vi "FMA1600A Main.vi"() -> ()   [LabVIEW 2016]
uses:
  Type Definitions/FMA1600A Gas Type.ctl
  Type Definitions/FMA1600A Commands.ctl
  Alicat Gas Meter Driver/Sub-VIs/Data Cluster.ctl
  <vilib>/Utility/file.llb/Write To Spreadsheet File (string).vi
  <vilib>/Utility/file.llb/Write Delimited Spreadsheet (string).vi
panel:
  out "Data Cluster":T1
  in  "Use Data Save":bool
  in  "Scan Rate (mS)":u32=1000
  in  "file path (dialog if empty)":path=path "C:/Data/FMA1600A.csv"
  in  "Tab Control":enum32{"Page 1", "Page 2"}(tab)
  out "error out":errorcluster
  in  "Unit ID":string="A"
  in  "FMA1600A Commands":T2="*@="
  in  "Gas Type":T3="2"
  in  "stop":bool
  in  "VISA resource name":refnum<visa-resource-name>="COM3"
  # "Totalizer Timer"
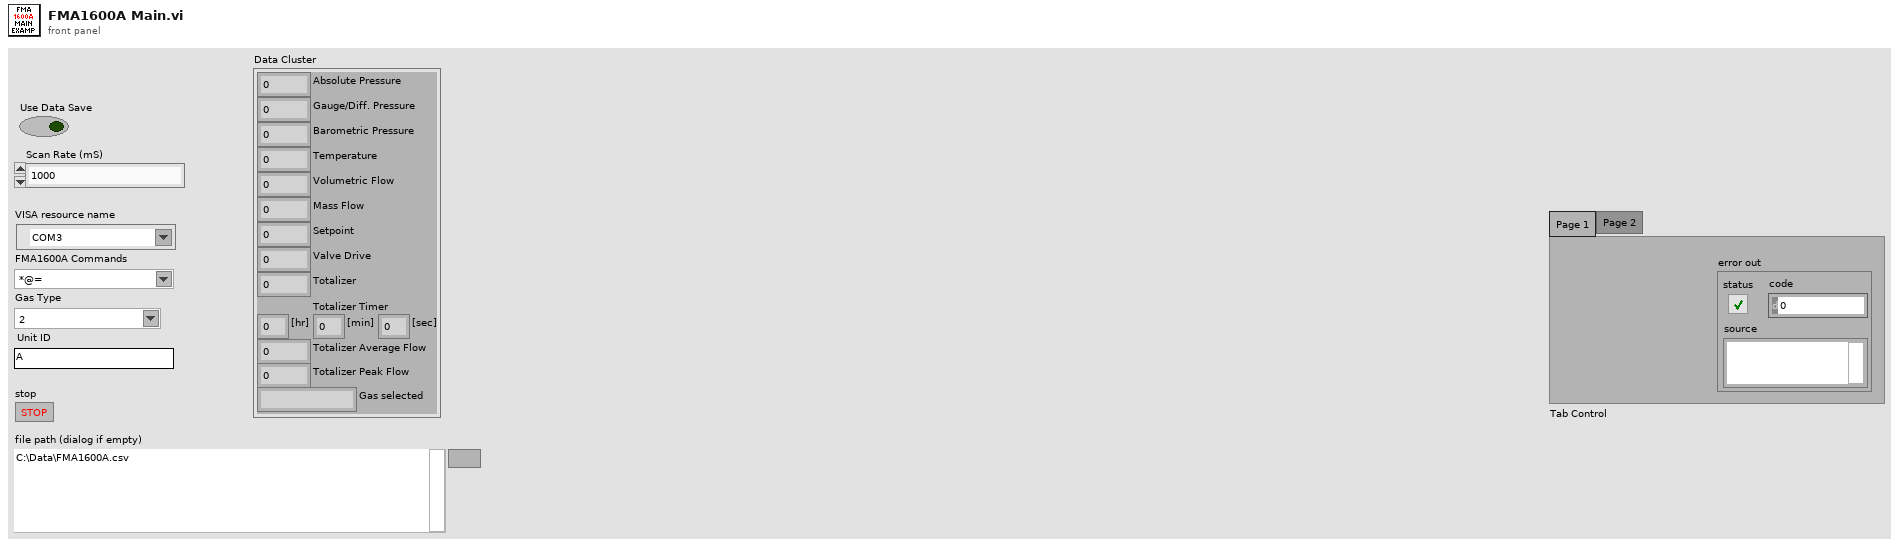
[diagram p1: front panel]
types:
  T1 = typedef "Data Cluster.ctl" = cluster{"Absolute Pressure":dbl, "Gauge/Diff. Pressure":dbl, "Barometric Pressure":dbl, "Temperature":dbl, "Volumetric Flow":dbl, "Mass Flow":dbl, "Setpoint":dbl, "Valve Drive":dbl, "Totalizer":dbl, "[hr]":dbl, "[min]":dbl, "[sec]":dbl, "Totalizer Average Flow":dbl, "Totalizer Peak Flow":dbl, "Gas selected":string}
  T2 = typedef "FMA1600A Commands.ctl" = string
  T3 = typedef "FMA1600A Gas Type.ctl" = string
  T4 = enum8{"2400", "9600", "19200", "38400", "57600", "115200", "Unknown"}
  T5 = typedef "Data Frame.ctl" = cluster{"Absolute Pressure":bool, "Gauge/Diff. Pressure":bool, "Barometric Pressure":bool, "Temperature":bool, "Volumetric":bool, "Mass":bool, "Setpoint":bool, "Valve Drive":bool, "Totalizer":bool, "Totalizer Timer":bool, "Totalizer Average Flow":bool, "Totalizer Peak Flow":bool, "Gas Selected":bool, "Tot. Timer Format":u16}
  T6 = typedef "FMA1600A Data.ctl" = cluster{"Pressure (PSIA)":dbl, "Temperature (°F)":dbl, "Vol. Flow (LPM)":dbl, "Mass Flow (SLPM)":dbl, "Gas Type":string, "Tot. Flow (Liters)":dbl, "Meter ID":string}
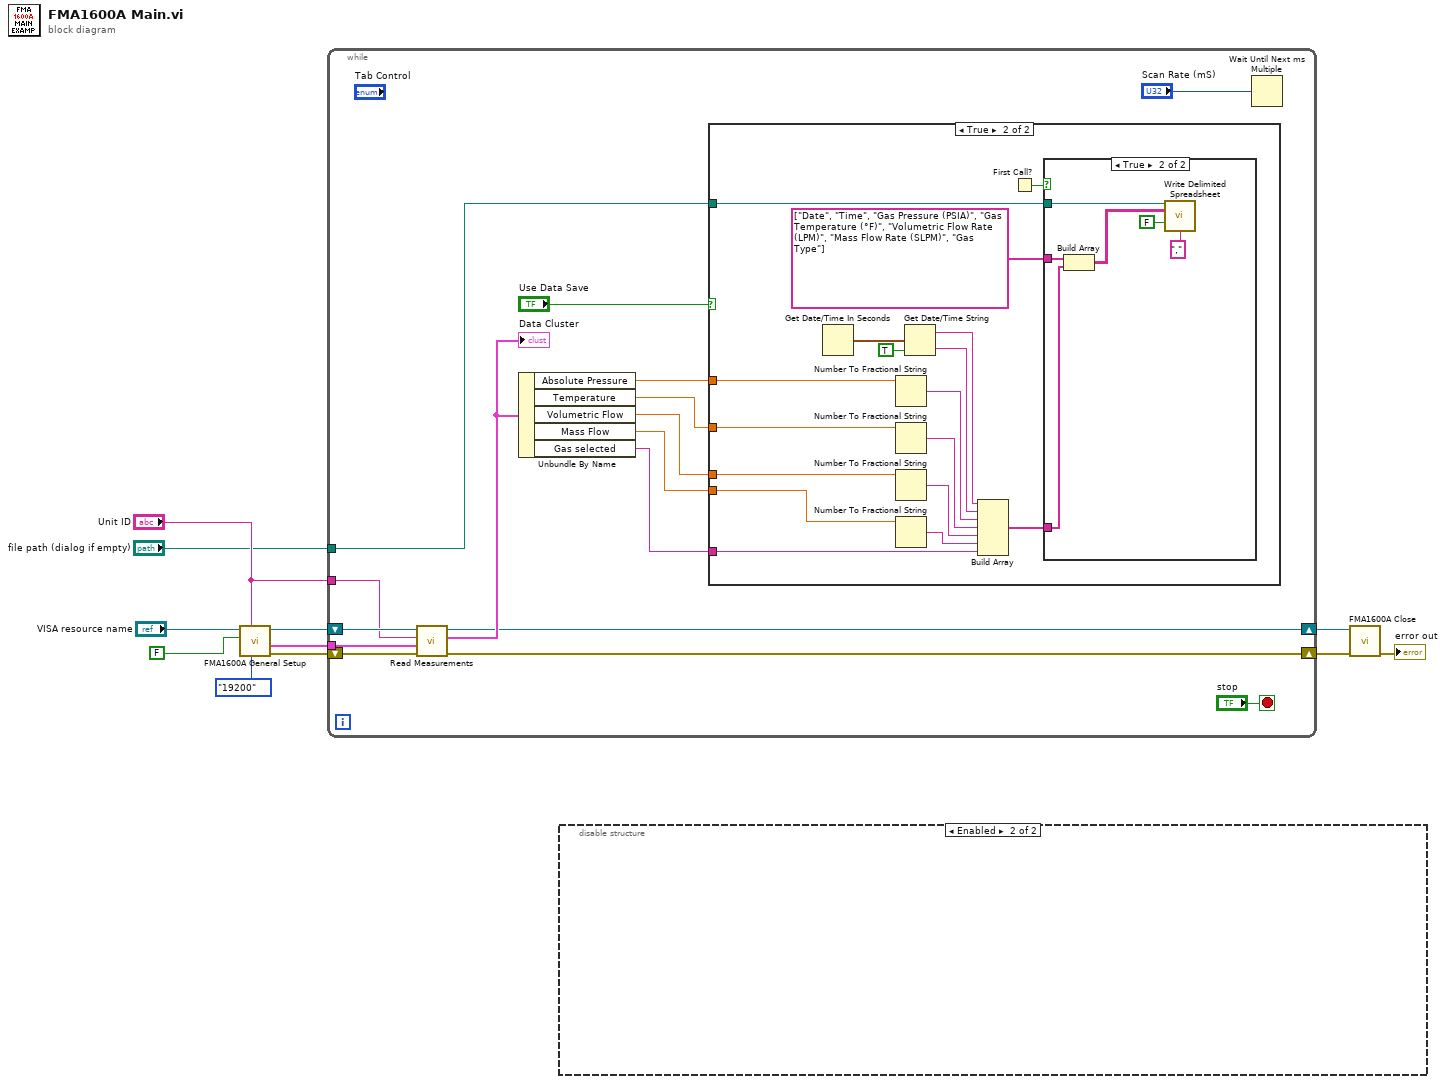
[diagram p0: block diagram]
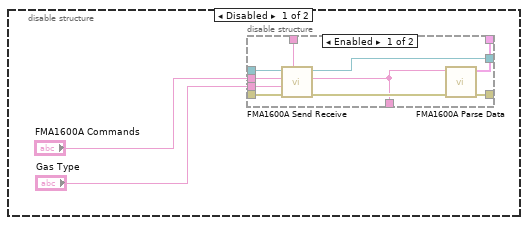
[diagram p2: hidden frame]
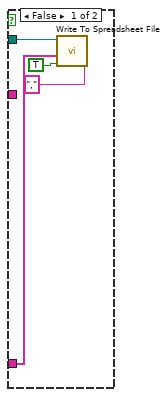
[diagram p5: hidden frame]
diagram:
  n1 = call "FMA1600A General Setup.vi"("Baud Rate"=T4."19200", "Unit ID"="Unit ID", "Set STP Register"=FALSE, "VISA Refnum in"="VISA resource name") -> ("error out"=w4:errorcluster, "Data Frame Format"=w2:T5, "VISA Refnum out"=w8:refnum<visa-resource-name>)  [unwired: 4 in, 1 out]
  n2 = while {
    shift-right: [w12] -> w9
    shift-left: w8 -> [w21]
    tunnel: "Unit ID" -> [w19]
    tunnel: "file path (dialog if empty)" -> [w25]
    shift-right: [w23] -> w11
    shift-left: w4 -> [w22]
    tunnel: w2 -> [w20]
    stop <- "stop" stop-if-true
    n3 = call "Read Measurements.vi"("error in"=w22, "Data Frame Format In"=w20, "Unit ID (A)"=w19, "VISA Session In"=w21) -> ("error out"=w23:errorcluster, "Data Cluster"=w18:T1, "VISA Session Out"=w12:refnum<visa-resource-name>)  [unwired: 5 out]
    "Data Cluster" <- w18
    n4 = Unbundle By Name(w18) -> ("Absolute Pressure"=w17:dbl, "Temperature"=w16:dbl, "Volumetric Flow"=w15:dbl, "Mass Flow"=w14:dbl, "Gas selected"=w13:string)
    n5 = case shown="True" "Use Data Save" {
      tunnel: w25 -> [_ w33]
      tunnel: w17 -> [_ w32]
      tunnel: w16 -> [_ w31]
      tunnel: w15 -> [_ w30]
      tunnel: w14 -> [_ w29]
      tunnel: w13 -> [_ w28]
      frame False {
      }
      frame True {
        n6 = Get Date/Time In Seconds() -> (seconds since 1Jan1904=w44:timestamp)
        n7 = Number To Fractional String(number=w32) -> (F-format string=w43:string)  [unwired: 3 in]
        n8 = Number To Fractional String(number=w31) -> (F-format string=w42:string)  [unwired: 3 in]
        n9 = Number To Fractional String(number=w30) -> (F-format string=w41:string)  [unwired: 3 in]
        n10 = Number To Fractional String(number=w29) -> (F-format string=w40:string)  [unwired: 3 in]
        n11 = Get Date/Time String(seconds (now)=w44, want seconds? (F)=TRUE) -> (date string=w36:string, time string=w37:string)  [unwired: 1 in]
        n12 = Build Array(w36, w37, w43, w42, w41, w40, w28) -> (w39:string[])
        n13 = First Call?() -> (First Call?: T/F=w34:bool)
        n14 = case shown="True" w34 {
          tunnel: w39 -> [w46 w54]
          tunnel: string[] ["Date", "Time", "Gas Pressure (PSIA)", "Gas Temperature (°F)", "Volumetric Flow Rate (LPM)", "Mass Flow Rate (SLPM)", "Gas Type"] -> [_ w53]
          tunnel: w33 -> [w47 w51]
          frame False {
            n15 = call-poly <vilib>:"Write To Spreadsheet File.vi"("delimiter (\\t)"="," ("delimiter (\\t)"), "append to file? (new file:F)"=TRUE, "1D data"=w46, "file path (dialog if empty)"=w47) -> ()  [unwired: 4 in, 1 out]
          }
          frame True {
            n16 = Build Array(w53, w54) -> (w52:string[][])
            n17 = call-poly <vilib>:"Write Delimited Spreadsheet.vi"("file path (dialog if empty)"=w51, "2D data"=w52, "append to file? (new file:F)"=FALSE, "delimiter (\\t)"="," ("delimiter (\\t)")) -> ()  [unwired: 10 in, 2 out]
          }
        }
      }
    }
    n18 = Wait Until Next ms Multiple(millisecond multiple="Scan Rate (mS)") -> ()  [unwired: 1 out]
  }
  n19 = disable-structure shown="Enabled" {
    frame Disabled {
      n20 = disable-structure shown="Enabled" {
        disable-tunnel: [w69 w70] -> w55
        disable-tunnel: "FMA1600A Commands" -> [w68 _]
        disable-tunnel: [w66 w71] -> _
        disable-tunnel: [w65 _] -> _
        disable-tunnel: "Gas Type" -> [w64 _]
        disable-tunnel: [w63 _] -> w58
        disable-tunnel: [w62 _] -> _
        disable-tunnel: [w61 w70] -> _
        disable-tunnel: [w60 w71] -> w59
        frame Enabled {
          n21 = call "FMA1600A Send Receive.vi"("Unit ID"=w63, "error in (no error)"=w60, "Gas Type"=w64, "FMA1600A Commands"=w68, "VISA Refnum in"=w69) -> ("error out"=w67:errorcluster, "Raw FMA1600A Data"=w65:string, "VISA Refnum out"=w61:refnum<visa-resource-name>)  [unwired: 4 in]
          n22 = call "FMA1600A Parse Data.vi"("Error In"=w67, "Raw FMA1600A Data"=w65) -> ("Error Out"=w66:errorcluster, "FMA1600A Gas Data"=w62:T6)  [unwired: 7 in]
        }
        frame Disabled {
        }
      }
    }
    frame Enabled {
    }
  }
  n23 = call "FMA1600A Close.vi"("error in (no error)"=w11, "VISA Refnum in"=w9) -> ("error out"=→"error out":errorcluster)  [unwired: 9 in]
